vi "Disconnect from Target.vi"(8 "error in (no error)":errorcluster, 11 "Program Data":T1={"Measurements"={"Channel 0"="Channel 0", "RMS 0"="RMS:", "Vp-p 0"="Vp-p:", "Freq 0"="Freq:", "Channel 1"="Channel 1", "RMS 1"="RMS:", "Vp-p 1"="Vp-p:", "Freq 1"="Freq:", "Cursors"="Channel 0", "C1"="Channel 0", "C2"="Channel 0", "dT"="Channel 0"}, "C1"={"Name"="", "X"=0.0, "Y"=0.0}, "C2"={"Name"="", "X"=0.0, "Y"=0.0}, "Com"={"Connection Info"={"connection ID"=refnum, "meta data"=[]}, "Connected?"=FALSE, "IP"=""}, "Continuous?"=FALSE, "Scope Data"={"AI0"=[], "AI1"=[]}, "Wave Parameters"={"Frequency (Hz)"=5.0, "Phase offset (deg)"=0.0, "Vpeak (V)"=5.0, "Offset (V)"=0.0, "Waveform"=enum."Sine", "Channel"=enum."CH0"}, "Acquire?"=FALSE, "Measure Ref"=refnum, "CH0"={"Channel"=enum."AI 0", "Enable"=FALSE, "Volts/Div"=0, "Vertical Position (Div)"=0.0}, "CH1"={"Channel"=enum."AI 0", "Enable"=FALSE, "Volts/Div"=0, "Vertical Position (Div)"=0.0}, "CH0 Params"={"V/Div"=0.0, "Units"=""}, "CH1 Params"={"V/Div"=0.0, "Units"=""}, "Time"={"Time/Div"=0.0}, "dT"=0.0, "FGen"={"Offset (V)"=0.0, "Enable Sweep"=FALSE, "Start Frequency (Hz)"=0.0, "Stop Frequency (Hz)"=0.0, "Step (Hz)"=0.0, "Step Interval (ms)"=0.0, "Current Freq (Hz)"=0.0, "Run"=FALSE}} {"Time"."Time/Div" min=0.0 max=16.0 step=1.0 scale=0.0..12.0; "CH1"."Vertical Position (Div)" min=-5.0 max=5.0 step=0.1 scale=-5.0..5.0; "CH1"."Volts/Div" min=0 max=8 step=1 scale=0.0..8.0; "CH0"."Vertical Position (Div)" min=-5.0 max=5.0 step=0.1 scale=-5.0..5.0; "CH0"."Volts/Div" min=0 max=8 step=1 scale=0.0..8.0; "Wave Parameters"."Phase offset (deg)" format="%#_6p"; "Wave Parameters"."Frequency (Hz)" format="%#_6p"}) -> (0 "error out":errorcluster, 3 "Program Data out":T1={"Measurements"={"Channel 0"="Channel 0", "RMS 0"="RMS:", "Vp-p 0"="Vp-p:", "Freq 0"="Freq:", "Channel 1"="Channel 1", "RMS 1"="RMS:", "Vp-p 1"="Vp-p:", "Freq 1"="Freq:", "Cursors"="Channel 0", "C1"="Channel 0", "C2"="Channel 0", "dT"="Channel 0"}, "C1"={"Name"="", "X"=0.0, "Y"=0.0}, "C2"={"Name"="", "X"=0.0, "Y"=0.0}, "Com"={"Connection Info"={"connection ID"=refnum, "meta data"=[]}, "Connected?"=FALSE, "IP"=""}, "Continuous?"=FALSE, "Scope Data"={"AI0"=[], "AI1"=[]}, "Wave Parameters"={"Frequency (Hz)"=5.0, "Phase offset (deg)"=0.0, "Vpeak (V)"=5.0, "Offset (V)"=0.0, "Waveform"=enum."Sine", "Channel"=enum."CH0"}, "Acquire?"=FALSE, "Measure Ref"=refnum, "CH0"={"Channel"=enum."AI 0", "Enable"=FALSE, "Volts/Div"=0, "Vertical Position (Div)"=0.0}, "CH1"={"Channel"=enum."AI 0", "Enable"=FALSE, "Volts/Div"=0, "Vertical Position (Div)"=0.0}, "CH0 Params"={"V/Div"=0.0, "Units"=""}, "CH1 Params"={"V/Div"=0.0, "Units"=""}, "Time"={"Time/Div"=0.0}, "dT"=0.0, "FGen"={"Offset (V)"=0.0, "Enable Sweep"=FALSE, "Start Frequency (Hz)"=0.0, "Stop Frequency (Hz)"=0.0, "Step (Hz)"=0.0, "Step Interval (ms)"=0.0, "Current Freq (Hz)"=0.0, "Run"=FALSE}} {"Time"."Time/Div" min=0.0 max=16.0 step=1.0 scale=0.0..12.0; "CH1"."Vertical Position (Div)" min=-5.0 max=5.0 step=0.1 scale=-5.0..5.0; "CH1"."Volts/Div" min=0 max=8 step=1 scale=0.0..8.0; "CH0"."Vertical Position (Div)" min=-5.0 max=5.0 step=0.1 scale=-5.0..5.0; "CH0"."Volts/Div" min=0 max=8 step=1 scale=0.0..8.0; "Wave Parameters"."Phase offset (deg)" format="%#_6p"; "Wave Parameters"."Frequency (Hz)" format="%#_6p"})   [LabVIEW 2021]
uses:
  Controls/Program Data.ctl
  Controls/Measurements.ctl
  Controls/Channel Measurement String Control.ctl
  Controls/Cursor Info.ctl
  Controls/Communication Cluster.ctl
  <vilib>/NI/STM/TCP/TCP Connection Info.ctl
  <vilib>/NI/STM/SubVIs/MetaDataElement.ctl
  Scope Data.ctl
  Program Files (x86)/National Instruments/LabVIEW 2021/ProjectTemplates/Source/myRIO/Oscilloscope/myRIO v1.1/Real-Time/Controls/Wave Parameters.ctl
  Program Files (x86)/National Instruments/LabVIEW 2021/ProjectTemplates/Source/myRIO/Oscilloscope/myRIO v1.1/Real-Time/Controls/Waveform Enum.ctl
  Program Files (x86)/National Instruments/LabVIEW 2021/ProjectTemplates/Source/myRIO/Oscilloscope/myRIO v1.1/Real-Time/Controls/Channel Selector.ctl
  Controls/Channel Settings.ctl
  Controls/Analog Input Selector.ctl
  Controls/Knob.ctl
  Controls/Vertical Position.ctl
  Controls/Channel Parameters.ctl
  Controls/Time Selector.ctl
  Controls/Time Knob.ctl
  Controls/FGen Desktop Configuration.ctl
  <vilib>/NI/STM/TCP/Get Connection Reference (TCP).vi
  <vilib>/NI/STM/NI STM.lvlib
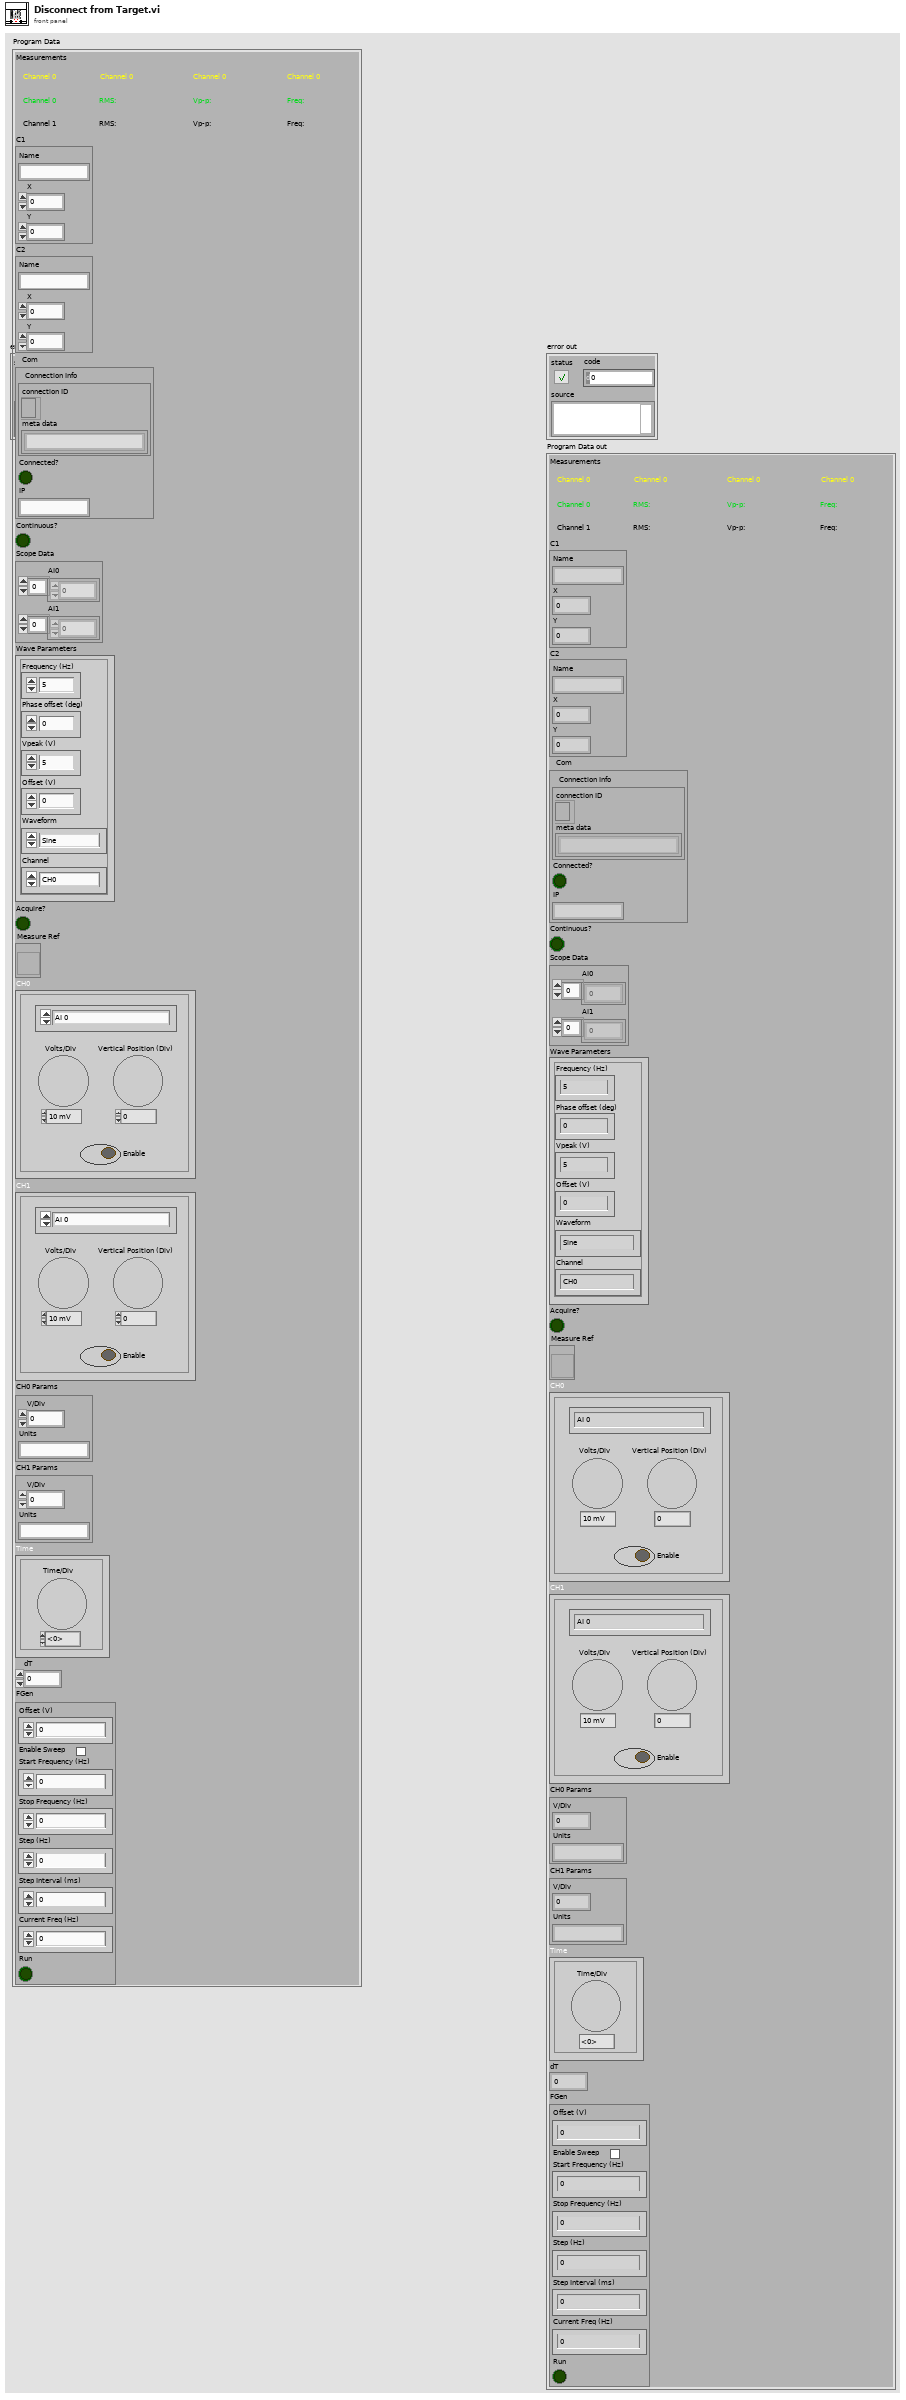
[diagram p1: front panel]
types:
  T1 = typedef "Program Data.ctl" = cluster{"Measurements":T2, "C1":T4, "C2":T4, "Com":T5, "Continuous?":bool, "Scope Data":T8, "Wave Parameters":T9, "Acquire?":bool, "Measure Ref":refnum<vi>, "CH0":T12, "CH1":T12, "CH0 Params":T16, "CH1 Params":T16, "Time":T17, "dT":dbl, "FGen":T19}
  T2 = typedef "Measurements.ctl" = cluster{"Channel 0":T3, "RMS 0":T3, "Vp-p 0":T3, "Freq 0":T3, "Channel 1":T3, "RMS 1":T3, "Vp-p 1":T3, "Freq 1":T3, "Cursors":T3, "C1":T3, "C2":T3, "dT":T3}
  T3 = typedef "Channel Measurement String Control.ctl" = string
  T4 = typedef "Cursor Info.ctl" = cluster{"Name":string, "X":dbl, "Y":dbl}
  T5 = typedef "Communication Cluster.ctl" = cluster{"Connection Info":T6, "Connected?":bool, "IP":string}
  T6 = typedef "NI STM.lvlib/TCP Connection Info.ctl" = cluster{"connection ID":refnum<k5>, "meta data":T7[]}
  T7 = typedef "NI STM.lvlib/MetaDataElement.ctl" = string
  T8 = typedef "Scope Data.ctl" = cluster{"AI0":dbl[], "AI1":dbl[]}
  T9 = typedef "Wave Parameters.ctl" = cluster{"Frequency (Hz)":dbl, "Phase offset (deg)":dbl, "Vpeak (V)":dbl, "Offset (V)":dbl, "Waveform":T10, "Channel":T11}
  T10 = typedef "Waveform Enum.ctl" = enum16{"Sine", "Square"}
  T11 = typedef "Channel Selector.ctl" = enum16{"CH0", "CH1"}
  T12 = typedef "Channel Settings.ctl" = cluster{"Channel":T13, "Enable":bool, "Volts/Div":T14, "Vertical Position (Div)":T15}
  T13 = typedef "Analog Input Selector.ctl" = enum16{"AI 0", "AI 1"}
  T14 = typedef "Knob.ctl" = i32
  T15 = typedef "Vertical Position.ctl" = dbl
  T16 = typedef "Channel Parameters.ctl" = cluster{"V/Div":dbl, "Units":string}
  T17 = typedef "Time Selector.ctl" = cluster{"Time/Div":T18}
  T18 = typedef "Time Knob.ctl" = dbl
  T19 = typedef "FGen Desktop Configuration.ctl" = cluster{"Offset (V)":dbl, "Enable Sweep":bool, "Start Frequency (Hz)":dbl, "Stop Frequency (Hz)":dbl, "Step (Hz)":dbl, "Step Interval (ms)":dbl, "Current Freq (Hz)":dbl, "Run":bool}
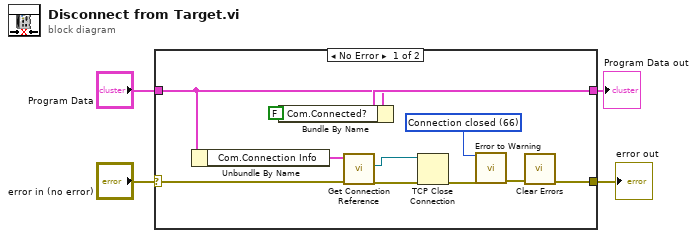
[diagram p0: block diagram]
diagram:
  n1 = case shown="No Error" "error in (no error)" {
    selector: "error in (no error)" -> [w11 w17]
    tunnel: "Program Data" -> [w6 w16]
    tunnel: [w9 w17] -> w3
    tunnel: [w8 w16] -> w1
    frame No Error {
      w12 = 66 items=["No Error", "Argument Error", "Memory Full", "Out of Zone", "End of File", "File Already Open", "Generic File IO Error", "File Not Found", "File Permission Error", "Disk Full", "Duplicate Path", "Too Many Files Open", "Not Enabled", "Resource File Not Found", "Cannot Add Resource", "Resource Not Found", "Image Not Found", "Image Memory Error", "Pen Does Not Exist", "Config Bad Type", "Config Token Not Found", "Config Parse Error", "Config Memory Error", "Bad External Code Format", "Bad External Code Offset", "External Code Not Present", "Null Window", "Destroy Window Mixup", "Null Menu", "Print Aborted", "Bad Print Record", "Print Driver Error", "Windows Error During Print", "Memory Error During Print", "Print Dialog Error", "Generic Print Error", "Invalid Device Refnum", "Device Not Found", "Device Parameter Error", "Device Unit Error", "Can't Open Device", "Device Call Aborted", "Generic Error", "Cancelled By User", "Object ID Too Low", "Object ID Too High", "Object Not In Heap", "Unknown Heap", "Bad DefProc ID", "DefProc Not In Table", "Message Out Of Range", "Null Method", "Unknown Message", "Manager Call Not Supported", "Bad address", "Connection In progress", "Connection timed out", "Connection is already in progress", "Network attribute not supported", "Network error", "Address in use", "System out of memory", "Connection aborted", "Connection refused", "Connection is not connected", "Connection is already connected", "Connection closed", "Initialize error (interapplication manager)", "Bad occurrence", "Wait on unbound occurrence handler", "Occurrence queue overflow", "Bad path", "Semaphore not signaled", "Unrecognized type (interapplication manager)"] ("1st Error to Convert")
      n2 = Unbundle By Name(w6) -> ("Com.Connection Info"=w5:T6)
      n3 = Bundle By Name(cluster=w6, "Com.Connected?"=FALSE ("Connected?")) -> (w8:T1)
      n4 = call-poly <vilib>:"Get Connection Reference.vi"("error in"=w11, "connection info in"=w5) -> ("error out"=w15:errorcluster, "connection ID out"=w14:refnum<k5>)  [unwired: 8 out]
      n5 = TCP Close Connection(connection ID=w14, error in (no error)=w15) -> (error out=w13:errorcluster)  [unwired: 2 out]
      n6 = call <vilib>:"Error to Warning.vi"("1st Error to Convert"=w12, "error in"=w13) -> ("warning out"=w10:errorcluster)  [unwired: 3 in, 10 out]
      n7 = call <vilib>:"Clear Errors.vi"("error in (no error)"=w10) -> ("error out"=w9:errorcluster)  [unwired: 5 in, 1 out]
    }
    frame Error {
    }
  }
  "error out" <- w3
  "Program Data out" <- w1
